vi "CNR Hessian diagonal scaling.vi"(7 "parameters":dbl[](array[numeric]), 10 "gradient":dbl[](array[numeric]), 11 "Hessian":T1) -> (1 "D":dbl[](array[numeric]), 2 "scaled gradient":dbl[](array[numeric]), 3 "scaled Hessian":T1, 5 "scaled parameters":dbl[](array[numeric]))   [LabVIEW 2014, in "NI_Gmath.lvlib"]
uses:
  NI_Gmath.lvlib
  RealMatrix.ctl
  NI_Matrix.lvlib
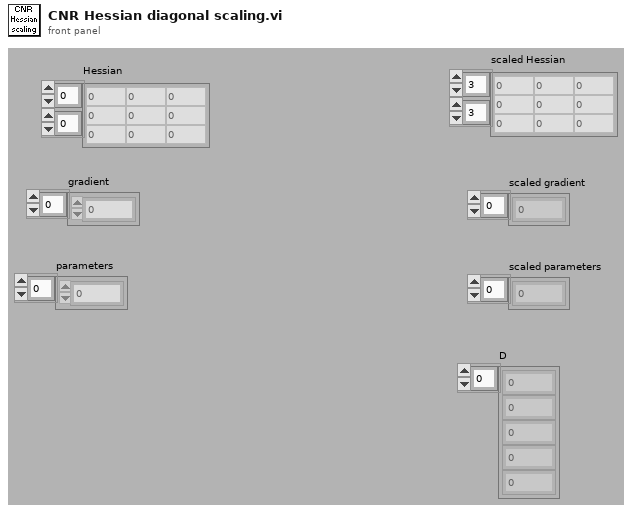
[diagram p1: front panel]
types:
  T1 = typedef "NI_Matrix.lvlib/RealMatrix.ctl" = dbl[][]
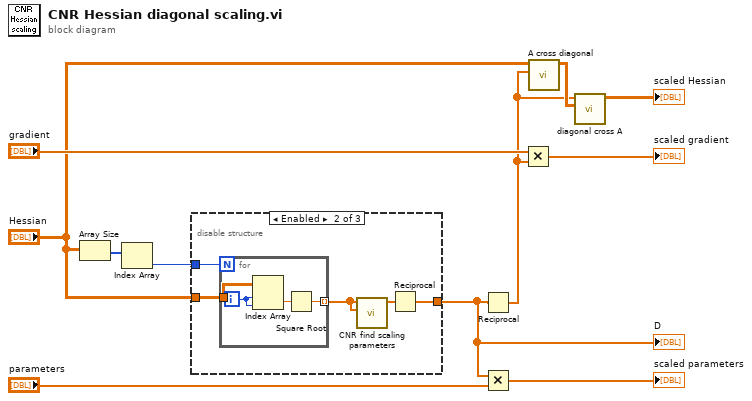
[diagram p0: block diagram]
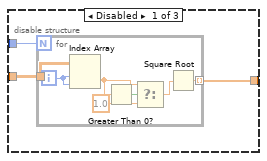
[diagram p2: hidden frame]
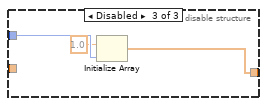
[diagram p3: hidden frame]
diagram:
  n1 = Array Size(array="Hessian") -> (size(s)=w11:i32[])
  n2 = Index Array(array=w11) -> (element=w10:i32)  [unwired: 1 in]
  n3 = disable-structure shown="Enabled" {
    disable-tunnel: w10 -> [w14 w26 w33]
    disable-tunnel: "Hessian" -> [w13 w25 _]
    disable-tunnel: [w12 w22 w31] -> w3
    frame Disabled {
      n4 = for {
        N: w14 -> [_]
        tunnel: w13 -> [w20]
        tunnel: [w19] -> w12 mode=indexing
        i -> [w21]
        n5 = Index Array(array=w20, index (row)=w21, index (col)=w21) -> (element=w16:dbl)
        n6 = Greater Than 0?(x=w16) -> (x > 0?=w18:bool)
        n7 = Select(t=w16, s=w18, f=1.0) -> (s? t:f=w15:dbl)
        n8 = Square Root(x=w15) -> (sqrt(x)=w19:dbl)
      }
    }
    frame Enabled {
      n9 = for {
        N: w26 -> [_]
        tunnel: w25 -> [w29]
        tunnel: [w28] -> w23 mode=indexing
        i -> [w30]
        n10 = Index Array(array=w29, index (row)=w30, index (col)=w30) -> (element=w27:dbl)
        n11 = Square Root(x=w27) -> (sqrt(x)=w28:dbl)
      }
      n12 = call "CNR find scaling parameters.vi"("parameters"=w23, "old parameter scale factors"=w23) -> ("parameter scale factors"=w24:dbl[])  [unwired: 9 in]
      n13 = Reciprocal(x=w24) -> (1/x=w22:dbl[])
    }
    frame Disabled {
      n14 = Initialize Array(1.0 ("element"), w33) -> (w31:dbl[])
    }
  }
  "D" <- w3
  n15 = Reciprocal(x=w3) -> (1/x=w6:dbl[])
  n16 = Multiply(x=w3, y="parameters") -> (x*y=→"scaled parameters":dbl[])
  n17 = Multiply(x="gradient", y=w6) -> (x*y=→"scaled gradient":dbl[])
  n18 = call "A cross diagonal.vi"("diagonal"=w6, "A"="Hessian") -> ("Axdiagonal"=w7:T1)  [unwired: 9 in]
  n19 = call "diagonal cross A.vi"("A"=w7, "diagonal"=w6) -> ("diagonalxA"=→"scaled Hessian":T1)  [unwired: 9 in]
